vi "Launch Live Report Viewer.vi"(8 "error in":errorcluster, 11 "TDMS in":refnum<class "TDMS.lvclass">) -> (0 "error out":errorcluster, 3 "TDMS out":refnum<class "TDMS.lvclass">)   [LabVIEW 2019, in "TDMS.lvlib" / "TDMS.lvclass"]
doc: "This is a wrapper function to provide asynchronous VI lauching of the live report viewer. \n\nAsynchronous launching is critical because it allows data capture/creation and update to continue in the background while the user is analyzing the data in real time. \n\nTo launch asynchronously a strictly typed vi reference must be passed into the call asnychronously application tool. That cannot be done with the dynamically dispatched Read Live Report VI. However, a static dispatched wrapper such as this can call the child function dynamically after it has been called. That is the purpose of this wrapper."
uses:
  TDMS.lvclass
  <vilib>/Utility/LVLibp/NI_PackedLibraryUtility.lvlib
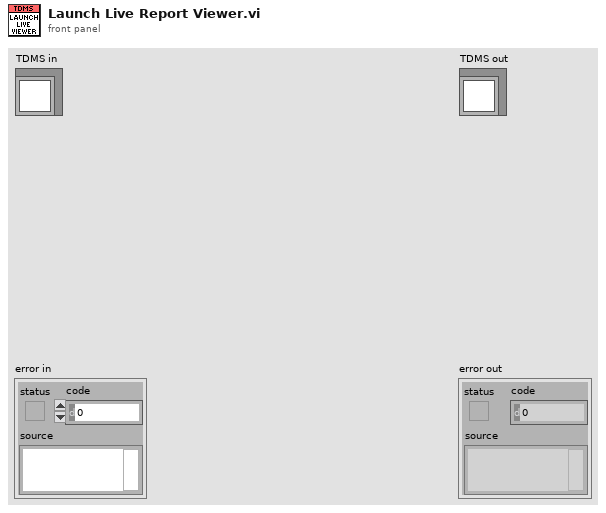
[diagram p1: front panel]
types:
  T1 = enum32{"Invalid", "Standard", "Closed", "Hidden", "Minimized", "Maximized"}
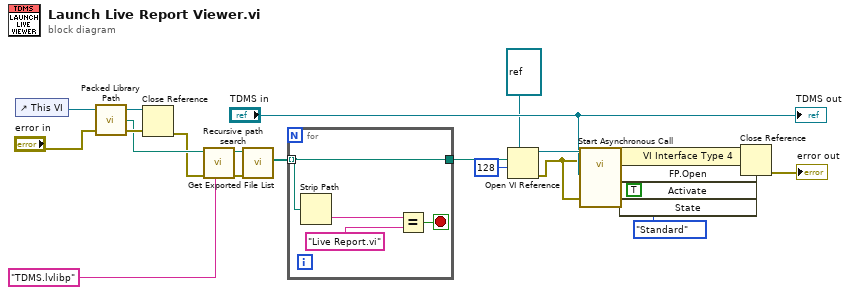
[diagram p0: block diagram]
diagram:
  n1 = control-ref of="This VI"() -> (w12:refnum<vi>)
  n2 = call <vilib>:"Packed Library Path.vi"("error in (no error)"="error in", "vi reference"=w12) -> ("error out"=w11:errorcluster, "packed library path"=w5:path, "vi reference out"=w10:refnum<vi>)  [unwired: 1 in]
  n3 = Close Reference(reference=w10, error in (no error)=w11) -> (error out=w1:errorcluster)
  n4 = call "Recursive path search.vi"("File name with extension"="TDMS.lvlibp", "error in"=w1, "Path"=w5) -> ("error out"=w2:errorcluster, "Path out"=w3:path)  [unwired: 7 in]
  n5 = call <vilib>:"Get Exported File List.vi"("error in (no error)"=w2, "packed library path"=w3) -> ("paths"=w8:path[])  [unwired: 7 in, 2 out]
  n6 = for {
    tunnel: w8 -> [w27] mode=indexing
    tunnel: [w27] -> w7
    stop <- w24 stop-if-true
    n7 = Strip Path(path=w27) -> (name=w25:string)  [unwired: 1 out]
    n8 = Equal?(x=w25, y="Live Report.vi") -> (x = y?=w24:bool)
  }
  n9 = Open VI Reference(type specifier VI Refnum (for type only)=refnum<vi> refnum, vi path=w7, options=128) -> (vi reference=w23:refnum<vi>, error out=w13:errorcluster)  [unwired: 3 in]
  n10 = call-by-ref "Start Asynchronous Call"(reference=w23, error in=w13, "error in"=w13, "TDMS in"="TDMS in") -> (reference out=w22:refnum<vi>, error out=w21:errorcluster)  [unwired: 8 in, 2 out]
  n11 = invoke class="VI Interface Type 4" method="FP.Open"(reference=w22, error in=w21, "Activate"=TRUE ("Activate?"), "State"=T1."Standard") -> (reference out=w18:refnum<vi>, error out=w17:errorcluster)  [unwired: 1 in, 3 out]
  n12 = Close Reference(reference=w18, error in (no error)=w17) -> (error out=→"error out":errorcluster)
  "TDMS out" <- "TDMS in"
